vi "qNAV.vi"(0 "System no.":i32=1 min=1 max=4 step=1, 1 "Board":i32=1 min=1 max=5 step=1, 5 "error in":errorcluster) -> (14 "Number of readings":i32, 19 "error out":errorcluster)   [LabVIEW 2026]
doc: "Returns averaging-count setting (used for analog readings)."
uses:
  Communication/Syntax.ctl
  Communication/Global1.vi
panel:
  # "Returns averaging-count setting (used for analog readings)."
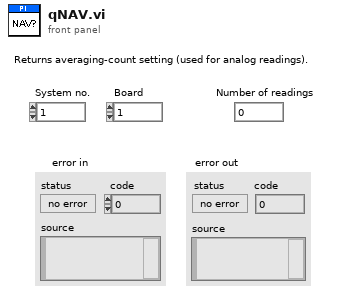
[diagram p1: front panel]
types:
  T1 = typedef "Syntax.ctl" = enum16{"GCS 1.0", "GCS 2.0", "GCS 3.0"}
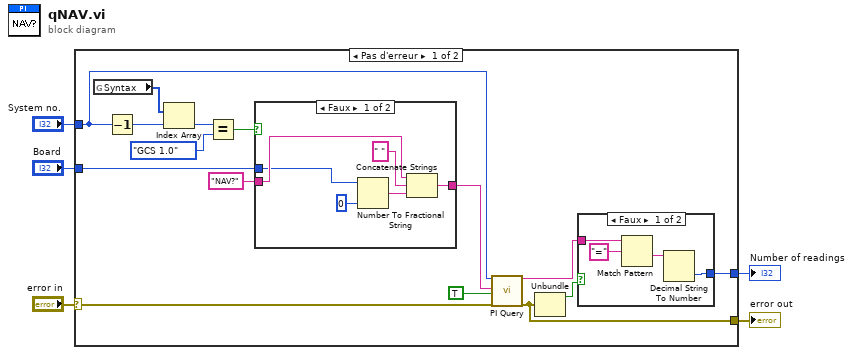
[diagram p0: block diagram]
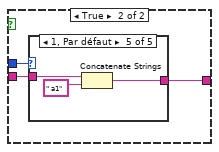
[diagram p2: hidden frame]
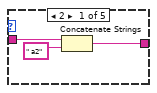
[diagram p3: hidden frame]
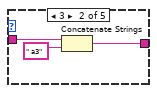
[diagram p4: hidden frame]
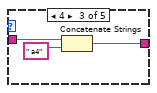
[diagram p5: hidden frame]
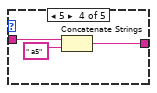
[diagram p6: hidden frame]
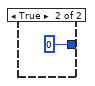
[diagram p7: hidden frame]
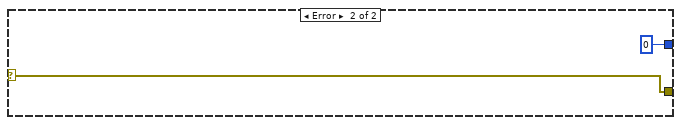
[diagram p8: hidden frame]
diagram:
  n1 = case shown="Pas d'erreur" "error in" {
    selector: "error in" -> [w9 w51]
    tunnel: [w19 0] -> w5
    tunnel: [w8 w51] -> w4
    tunnel: "Board" -> [w17 _]
    tunnel: "System no." -> [w10 _]
    frame No Error {
      n2 = global read "Global1.vi" "Syntax"() -> (w14:T1[])
      n3 = Decrement(x=w10) -> (x-1=w13:i32)
      n4 = Index Array(array=w14, index=w13) -> (element=w12:T1)
      n5 = Equal?(x=w12, y=Syntax."GCS 1.0") -> (x = y?=w11:bool)
      n6 = case shown="Faux" w11 {
        tunnel: w17 -> [w23 w29]
        tunnel: "NAV?" -> [w25 w28]
        tunnel: [w21 w27] -> w15
        frame False {
          n7 = Number To Fractional String(number=w23, precision (6)=i16 0) -> (F-format string=w22:string)  [unwired: 2 out]
          n8 = Concatenate Strings(w25, " ", w22) -> (w21:string)
        }
        frame True {
          n9 = case shown="1, Par défaut" w29 {
            tunnel: w28 -> [w32 w35 w38 w41 w44]
            tunnel: [w30 w33 w36 w39 w42] -> w27
            frame 2 {
              n10 = Concatenate Strings(w32, " a2" ("Substring")) -> (w30:string)
            }
            frame 3 {
              n11 = Concatenate Strings(w35, " a3" ("Substring")) -> (w33:string)
            }
            frame 4 {
              n12 = Concatenate Strings(w38, " a4" ("Substring")) -> (w36:string)
            }
            frame 5 {
              n13 = Concatenate Strings(w41, " a5" ("Substring")) -> (w39:string)
            }
            frame 1, Default {
              n14 = Concatenate Strings(w44, " a1" ("Substring")) -> (w42:string)
            }
          }
        }
      }
      n15 = call "PI Query.vi"("System no."=w10, "String to send"=w15, "Attach termination char.?"=TRUE ("Attach Linefeed?"), "error in"=w9) -> ("String read"=w7:string, "error out"=w8:errorcluster)  [unwired: 3 in, 11 out]
      n16 = Unbundle(w8) -> ("status"=w20:bool)  [unwired: 2 out]
      n17 = case shown="Faux" w20 {
        tunnel: w7 -> [w47 _]
        tunnel: [w48 0] -> w19
        frame False {
          n18 = Match Pattern(string=w47, regular expression="=") -> (after substring=w45:string)  [unwired: 4 out]
          n19 = Decimal String To Number(string=w45) -> (number=w48:i32)  [unwired: 3 out]
        }
        frame True {
        }
      }
    }
    frame Error {
    }
  }
  "error out" <- w4
  "Number of readings" <- w5
